vi "main.vi"() -> ()   [LabVIEW 2019]
panel:
  out "Picture":picture
  in  "function name":string="run_test"
  in  "module path":path=path "C:/Users/Computer/Documents/GitHub/MultiResUNet/load_model.py"
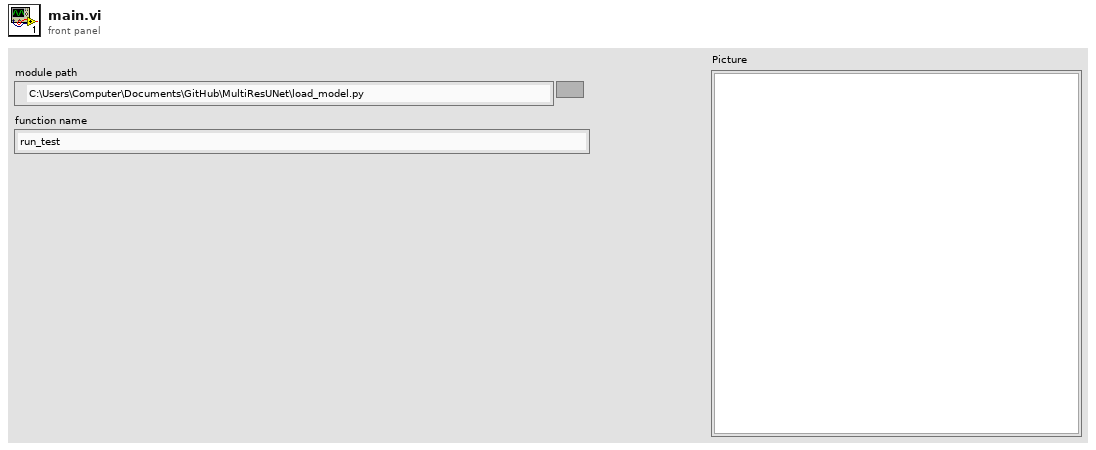
[diagram p1: front panel]
types:
  T1 = typedef "imagedata.ctl" = cluster{"image type":i32, "image depth":i32, "image":u8[], "mask":u8[], "colors":u32[], "Rectangle":cluster{"left":i16, "top":i16, "right":i16, "bottom":i16}}
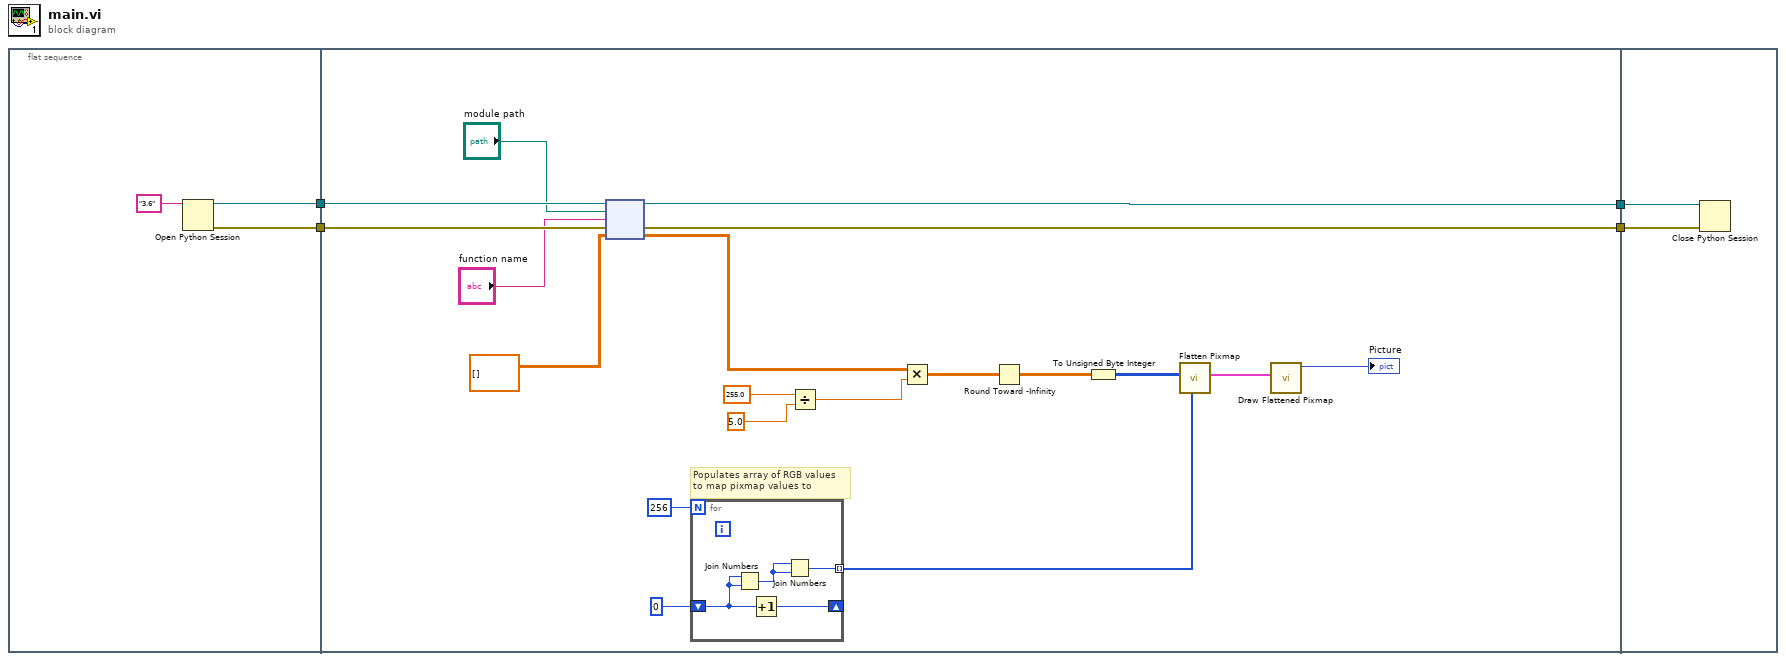
[diagram p0: block diagram]
diagram:
  n1 = flat-sequence {
    tunnel: [w7] -> w4
    tunnel: [w5] -> w2
    tunnel: w4 -> [w26]
    tunnel: [w25] -> w3
    tunnel: w2 -> [w24]
    tunnel: [w23] -> w1
    tunnel: w3 -> [w32]
    tunnel: w1 -> [w31]
    frame #0 {
      n2 = Open Python Session(python version="3.6" ("Python version")) -> (session out=w7:refnum<k35>, error out=w5:errorcluster)  [unwired: 2 in]
    }
    frame #1 {
      # "Populates array of RGB values\nto map pixmap values to"
      n3 = node(w26, "module path", "function name", w24, dbl[][] []) -> (w25:refnum<k35>, w23:errorcluster, w19:dbl[][])  [unwired: 2 out]
      n4 = for {
        N: 256 -> [_]
        tunnel: [w30] -> w8 mode=indexing
        shift-right: [w29] -> _
        shift-left: u8 0 -> [w27]
        n5 = Join Numbers(hi=w27, lo=w27) -> ((hi.lo)=w28:u16)
        n6 = Increment(x=w27) -> (x+1=w29:u8)
        n7 = Join Numbers(hi=w28, lo=w28) -> ((hi.lo)=w30:u32)
      }
      n8 = Divide(x=255.0, y=5.0) -> (x/y=w18:dbl)
      n9 = Multiply(x=w19, y=w18) -> (x*y=w15:dbl[][])
      n10 = Round Toward -Infinity(1:w15) -> (0:w14:dbl[][])
      n11 = To Unsigned Byte Integer(number=w14) -> (unsigned 8bit integer=w10:u8[][])
      n12 = call <vilib>:"Flatten Pixmap.vi"("colors"=w8, "8-bit pixmap"=w10) -> ("image data"=w11:T1)  [unwired: 9 in]
      n13 = call <vilib>:"Draw Flattened Pixmap.vi"("image data"=w11) -> ("new picture"=→"Picture":picture)  [unwired: 8 in]
    }
    frame #2 {
      n14 = Close Python Session(session in=w32, error in=w31) -> ()  [unwired: 1 out]
    }
  }
